vi "Request Command.vi"(8 "error in (no error)":errorcluster, 9 "Responses in":T1[](array[typedef]) {"Command" items=["Constant Speed Tracking"=8, "Echo"=55, "Error"=255, "Home"=1, "Limit Active"=9, "Manual Move Tracking"=10, "Move Absolute"=20, "Move at Constant Speed"=22, "Move Relative"=21, "Renumber"=2, "Restore Settings"=36, "Stop"=23]}, 10 "Request":T2={"Device Number"=0, "Command"=0, "Data"=0, "Response Count"=1} {"Command" items=["Echo"=55, "Home"=1, "Move Absolute"=20, "Move Relative"=21, "Move at Constant Speed"=22, "Renumber"=2, "Restore Settings"=36, "Stop"=23]}, 11 "VISA resource name":refnum<visa-resource-name>) -> (0 "error out":errorcluster, 1 "Responses out":T1[](array[typedef]) {"Command" items=["Constant Speed Tracking"=8, "Echo"=55, "Error"=255, "Home"=1, "Limit Active"=9, "Manual Move Tracking"=10, "Move Absolute"=20, "Move at Constant Speed"=22, "Move Relative"=21, "Renumber"=2, "Restore Settings"=36, "Stop"=23]}, 2 "First Response":T1 {"Command" items=["Constant Speed Tracking"=8, "Echo"=55, "Error"=255, "Home"=1, "Limit Active"=9, "Manual Move Tracking"=10, "Move Absolute"=20, "Move at Constant Speed"=22, "Move Relative"=21, "Renumber"=2, "Restore Settings"=36, "Stop"=23]}, 3 "VISA resource name out":refnum<visa-resource-name>)   [LabVIEW 2020, in "ZaberTSeries.lvlib"]
doc: "Sends a command and waits for a response. If the response is an error, sets error code -1074001617 and includes the Zaber error code in the message."
uses:
  ZaberTSeries.lvlib
  Request.ctl
  Response.ctl
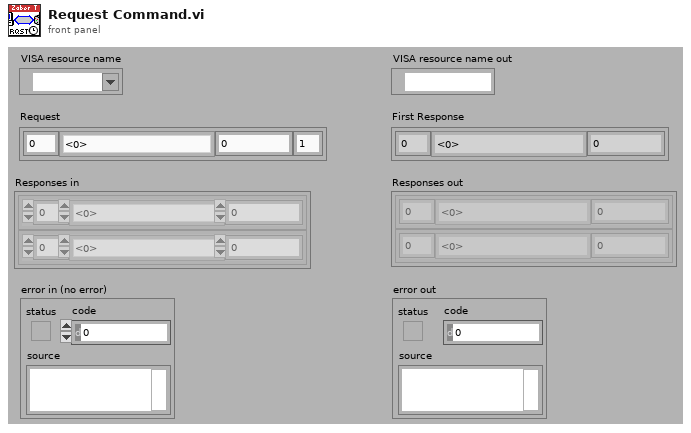
[diagram p1: front panel]
types:
  T1 = typedef "ZaberTSeries.lvlib/Response.ctl" = cluster{"Device Number":u8, "Command":u8, "Data":i32}
  T2 = typedef "ZaberTSeries.lvlib/Request.ctl" = cluster{"Device Number":u8, "Command":u8, "Data":i32, "Response Count":i32}
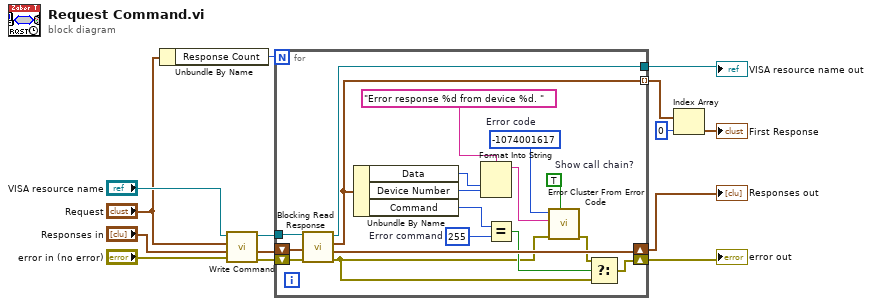
[diagram p0: block diagram]
diagram:
  n1 = Unbundle By Name("Request") -> ("Response Count"=w10:i32)
  n2 = call "Write Command.vi"("error in (no error)"="error in (no error)", "Responses in"="Responses in", "Request"="Request", "VISA resource name"="VISA resource name") -> ("error out"=w14:errorcluster, "Responses out"=w3:T1[], "VISA resource name out"=w6:refnum<visa-resource-name>)  [unwired: 5 in]
  n3 = for {
    N: w10 -> [_]
    tunnel: w6 -> [w30]
    shift-right: [w22] -> w9
    shift-left: w14 -> [w31]
    tunnel: [w29] -> w5
    shift-right: [w27] -> w2
    shift-left: w3 -> [w28]
    tunnel: [w26] -> w1 mode=indexing
    w24 = TRUE  # Show call chain?
    w25 = -1074001617  # Error code
    w32 = u8 255  # Error command
    n4 = call "Blocking Read Response.vi"("error in (no error)"=w31, "Responses in"=w28, "VISA resource name"=w30) -> ("error out"=w20:errorcluster, "Responses out"=w27:T1[], "Response"=w26:T1, "VISA resource name out"=w29:refnum<visa-resource-name>)  [unwired: 5 in]
    n5 = Unbundle By Name(w26) -> ("Data"=w17:i32, "Device Number"=w15:u8, "Command"=w16:u8)
    n6 = Format Into String(format string="Error response %d from device %d. " ("error message (\"\")"), w17, w15) -> (resulting string=w18:string)  [unwired: 2 in, 1 out]
    n7 = Equal?(x=w16, y=w32) -> (x = y?=w23:bool)
    n8 = call "Error Cluster From Error Code.vi"("show call chain? (False)"=w24, "error in (no error)"=w20, "error message (\"\")"=w18, "error code (0)"=w25) -> ("error out"=w19:errorcluster)  [unwired: 5 in]
    n9 = Select(t=w19, s=w23, f=w20) -> (s? t:f=w22:errorcluster)
  }
  "error out" <- w9
  "Responses out" <- w2
  "VISA resource name out" <- w5
  n10 = Index Array(array=w1, index=0) -> (element=→"First Response":T1)
